vi "PID parameters mMc.vi"(1 "Port":T1={"P type"=0, "reference"="", " Terminator "="\r\n", "Timeout"=300} {"Timeout" step=10; "P type" items=["none", "RS-232C"]}, 2 "PID in":cluster{"Kp":dbl, "Ki":dbl, "Kd":dbl}, 3 "error in (no error)":errorcluster, 4 "set/get":bool caption="set\n\n\nget", 5 "Controller #":string) -> (7 "PID out":cluster{"Kp":dbl, "Ki":dbl, "Kd":dbl}, 9 "error out":errorcluster)   [LabVIEW 2011]
panel:
  # "PID parameters"
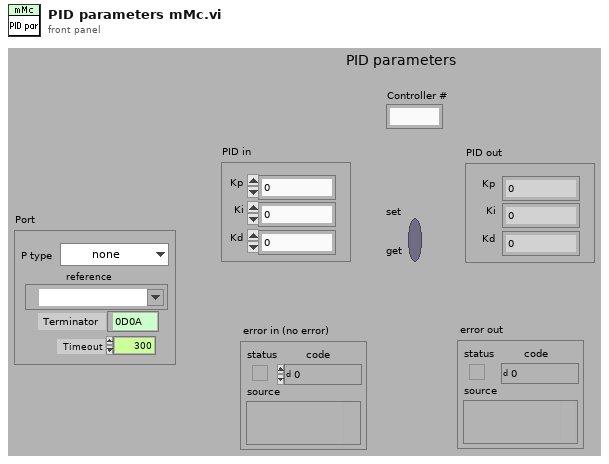
[diagram p1: front panel]
types:
  T1 = cluster{"P type":u16, "reference":refnum<visa-resource-name>, " Terminator ":string, "Timeout":i32}
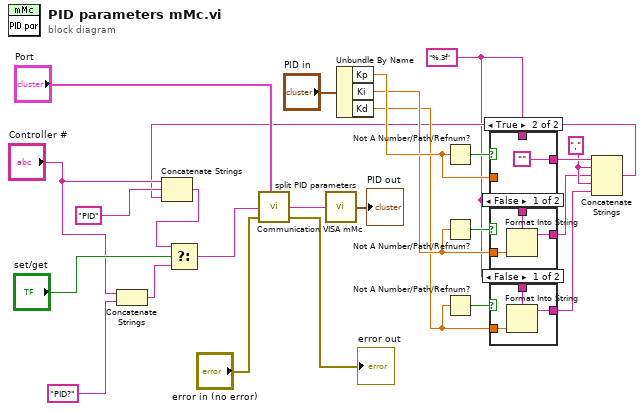
[diagram p0: block diagram]
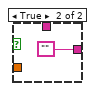
[diagram p2: hidden frame]
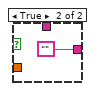
[diagram p3: hidden frame]
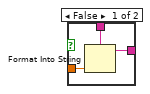
[diagram p4: hidden frame]
diagram:
  w1 = "%.3f" ("format string")
  w5 = ","
  n1 = Concatenate Strings("Controller #", "PID?") -> (w24:string)
  n2 = Unbundle By Name("PID in") -> ("Kp"=w12:dbl, "Ki"=w8:dbl, "Kd"=w7:dbl)
  n3 = Not A Number/Path/Refnum?(number/path/refnum=w12) -> (NaN/Path/Refnum?=w11:bool)
  n4 = Not A Number/Path/Refnum?(number/path/refnum=w8) -> (NaN/Path/Refnum?=w10:bool)
  n5 = Not A Number/Path/Refnum?(number/path/refnum=w7) -> (NaN/Path/Refnum?=w9:bool)
  n6 = case shown="True" w11 {
    tunnel: w12 -> [w28 _]
    tunnel: [w27 ""] -> w6
    tunnel: w1 -> [w26 _]
    frame False {
      n7 = Format Into String(format string=w26, w28) -> (resulting string=w27:string)  [unwired: 2 in, 1 out]
    }
    frame True {
    }
  }
  n8 = case shown="False" w10 {
    tunnel: w8 -> [w32 _]
    tunnel: [w31 ""] -> w4
    tunnel: w1 -> [w30 _]
    frame False {
      n9 = Format Into String(format string=w30, w32) -> (resulting string=w31:string)  [unwired: 2 in, 1 out]
    }
    frame True {
    }
  }
  n10 = case shown="False" w9 {
    tunnel: w7 -> [w36 _]
    tunnel: [w35 ""] -> w3
    tunnel: w1 -> [w34 _]
    frame False {
      n11 = Format Into String(format string=w34, w36) -> (resulting string=w35:string)  [unwired: 2 in, 1 out]
    }
    frame True {
    }
  }
  n12 = Concatenate Strings(w6, w5, w4, w5, w3) -> (w2:string)
  n13 = Concatenate Strings("Controller #", "PID", w2) -> (w22:string)
  n14 = Select(t=w22, s="set/get", f=w24) -> (s? t:f=w21:string)
  n15 = call "Communication VISA mMc.vi"("Port"="Port", "Command"=w21, "error in (no error)"="error in (no error)") -> ("Return"=w25:string, "error out"=→"error out":errorcluster)  [unwired: 3 in, 2 out]
  n16 = call "split PID parameters.vi"("string"=w25) -> ("PID out"=→"PID out":cluster{"Kp":dbl, "Ki":dbl, "Kd":dbl})  [unwired: 8 in]
